vi "Include ActorRef Queue Ref.vi"(8 "error in (no error)":errorcluster, 10 "NestedModule In":refnum<class "ModuleAbstract.lvclass">, 11 "LaunchingModule":refnum<class "ModuleAbstract.lvclass">) -> (0 "error out":errorcluster, 2 "NestedModule Out":refnum<class "ModuleAbstract.lvclass">)   [LabVIEW 2019, in "ModuleAbstract.lvlib" / "ModuleAbstract.lvclass"]
uses:
  ModuleAbstract.lvclass
  C:/Program Files (x86)/National Instruments/LabVIEW 2019/vi.lib/ActorFramework/Actor/Actor.lvclass
  ModuleAbstract.lvclass/ModuleAbstract.ctl
  Containers/ActorRefContainer/ActorRefContainer.lvclass
  <vilib>/ActorFramework/Actor/Actor.lvclass
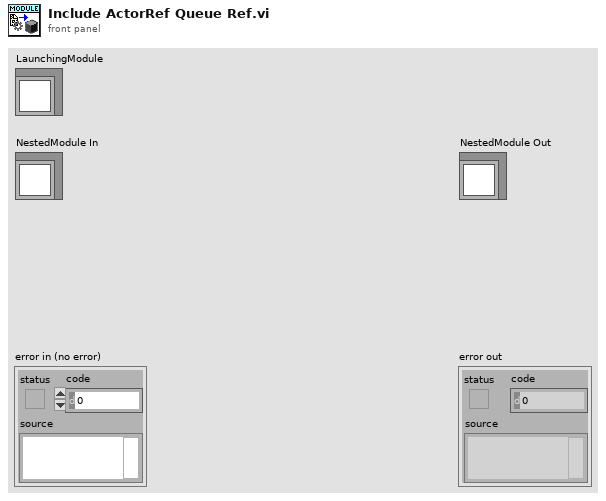
[diagram p1: front panel]
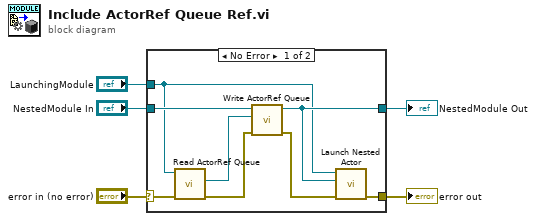
[diagram p0: block diagram]
diagram:
  n1 = case shown="No Error" "error in (no error)" {
    selector: "error in (no error)" -> [w11 w15]
    tunnel: [w8 w15] -> w4
    tunnel: [w7 w14] -> w2
    tunnel: "NestedModule In" -> [w13 w14]
    tunnel: "LaunchingModule" -> [w6 _]
    frame No Error {
      n2 = call "Read ActorRef Queue.vi"("error in (no error)"=w11, "ModuleAbstract in"=w6) -> ("error out"=w10:errorcluster, "ActorRef Queue"=w12:refnum<queue>)  [unwired: 7 in, 1 out]
      n3 = call "Write ActorRef Queue.vi"("error in (no error)"=w10, "ActorRef Queue"=w12, "ModuleAbstract in"=w13) -> ("error out"=w9:errorcluster, "ModuleAbstract out"=w7:refnum<class "ModuleAbstract.lvclass">)  [unwired: 7 in]
      n4 = call <vilib>:"Launch Nested Actor.vi"("error in (no error)"=w9, "Nested Actor"=w7, "Caller Actor in"=w6) -> ("error out"=w8:errorcluster)  [unwired: 6 in, 2 out]
    }
    frame Error {
    }
  }
  "error out" <- w4
  "NestedModule Out" <- w2
